vi "ReadWrite.ProcessData.Buffer.vi"(8 "error in":errorcluster, 9 "Offset":i32, 10 "Values":dbl[](array[numeric]), 11 "ReadWrite in":refnum<class "ReadWrite.lvclass">) -> (0 "error out":errorcluster, 3 "ReadWrite out":refnum<class "ReadWrite.lvclass">)   [LabVIEW 2024, in "VS Plugin Data Access Engine.lvlib" / "ReadWrite.lvclass"]
uses:
  ReadWrite.lvclass
  ReadWrite.lvclass/ReadWrite.ctl
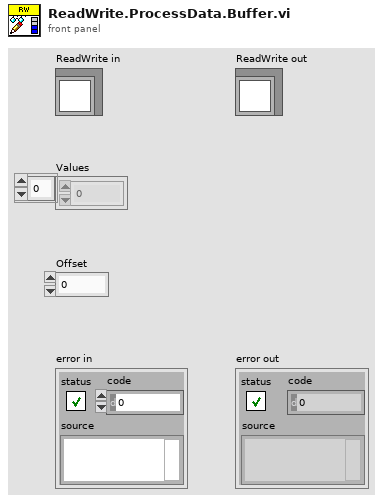
[diagram p1: front panel]
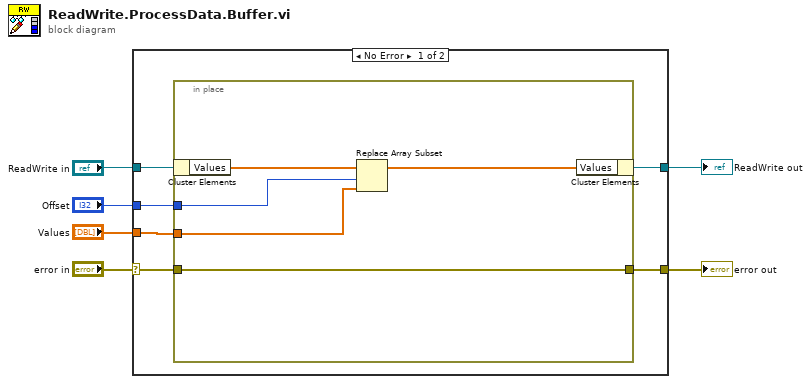
[diagram p0: block diagram]
diagram:
  n1 = case shown="No Error" "error in" {
    selector: "error in" -> [w12 w19]
    tunnel: [w11 w19] -> w5
    tunnel: [w9 w18] -> w1
    tunnel: "ReadWrite in" -> [w10 w18]
    tunnel: "Values" -> [w8 _]
    tunnel: "Offset" -> [w7 _]
    frame No Error {
      n2 = in-place {
        in-place-border: w12 -> [w17]
        in-place-border: w8 -> [w16]
        in-place-border: w7 -> [w15]
        in-place-border: [w17] -> w11
        n3 = in-place-cluster #1(w10) -> ("Values"=w14:dbl[])
        n4 = Replace Array Subset(array=w14, new element=w16, index=w15) -> (w13:dbl[])
        n5 = in-place-cluster #1("Values"=w13) -> (w9:refnum<class "ReadWrite.lvclass">)
      }
    }
    frame Error {
    }
  }
  "error out" <- w5
  "ReadWrite out" <- w1
